vi "Save Layout.vi"(5 "MultiPlotPanel in":refnum<class "MultiPlotPanel.lvclass">, 8 "error in (no error)":errorcluster, 10 "file extension":string, 11 "Loop data in":T1 {"PanelMap"."Data"."Plot Bounds (%)"."Bottom (%)" format="%.2f"; "PanelMap"."Data"."Plot Bounds (%)"."Top (%)" format="%.2f"; "PanelMap"."Data"."Plot Bounds (%)"."Right (%)" format="%.2f"; "PanelMap"."Data"."Plot Bounds (%)"."Left (%)" format="%.2f"}) -> (0 "error out":errorcluster, 1 "Valid save?":bool, 2 "Filename":string, 3 "Loop data out":T1 {"PanelMap"."Data"."Plot Bounds (%)"."Bottom (%)" format="%.2f"; "PanelMap"."Data"."Plot Bounds (%)"."Top (%)" format="%.2f"; "PanelMap"."Data"."Plot Bounds (%)"."Right (%)" format="%.2f"; "PanelMap"."Data"."Plot Bounds (%)"."Left (%)" format="%.2f"})   [LabVIEW 2021, in "MultiStokePlot.lvlib" / "MultiPlotPanel.lvclass"]
uses:
  Classes/MultiPlotPanel/MultiPlotPanel.lvclass
  Loop Data.ctl
  <vilib>/IlluminatedG/IG OOPanel/OOPanel/Manager/Manager.lvclass
  Panel Map.ctl
  Panel Map Data.ctl
  <userlib>/bjustice/RocketPlot/Classes/RocketPlotPanel/RocketPlotPanel.lvclass
  Window Position.ctl
  <vilib>/IlluminatedG/IG OOPanel/OOPanel/Panel/Panel Events.ctl
  <vilib>/IlluminatedG/IG OOPanel/OOPanel/Panel/Visbility Event Data.ctl
  <vilib>/IlluminatedG/IG OOPanel/OOPanel/Visibility State.ctl
  <vilib>/IlluminatedG/IG OOPanel/OOPanel/Close Reason.ctl
  Classes/MultiPlotPanel/MultiPlotPanel.lvclass/MultiPlotPanel.ctl
  Classes/BlueMultiPlotConfig/SinglePlotConfig.ctl
  <userlib>/bjustice/RocketPlot/TypeDefs/plot load data V2.ctl
  <userlib>/bjustice/RocketPlot/TypeDefs/plot properties V2.ctl
  <userlib>/bjustice/RocketPlot/TypeDefs/plot attributes V2.ctl
  <userlib>/bjustice/RocketPlot/TypeDefs/Plot scale axis properties.ctl
  <userlib>/bjustice/RocketPlot/TypeDefs/Plot general properties.ctl
  <userlib>/bjustice/RocketPlot/Classes/RocketPlotPanel/RocketPlotPanel.lvclass/RocketPlotPanel.ctl
  <userlib>/bjustice/RocketPlot/Classes/RocketPlotPanel/Read RocketPlotHandle.vi
  <userlib>/bjustice/RocketPlot/Classes/RocketPlotHandle/RocketPlotHandle.lvclass
  <userlib>/bjustice/RocketPlot/RocketPlot.lvlib
  <vilib>/IlluminatedG/IG OOPanel/OOPanel/OOPanel.lvlib
  <vilib>/IlluminatedG/IG OOPanel/OOPanel/Panel/Panel.lvclass
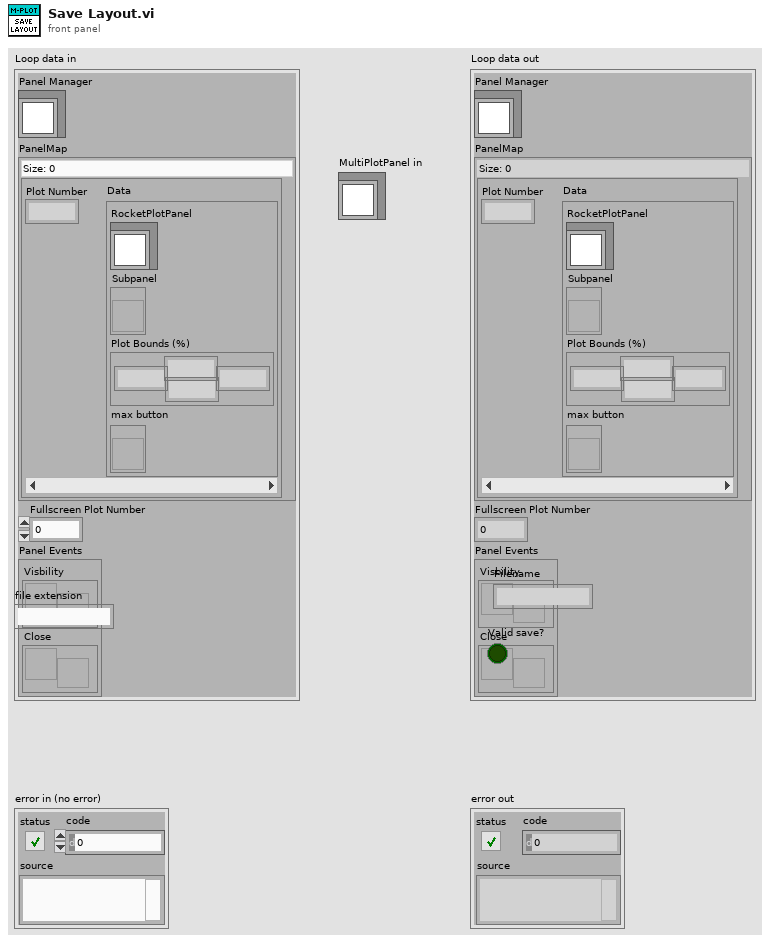
[diagram p1: front panel]
types:
  T1 = typedef "MultiStokePlot.lvlib/MultiPlotPanel.lvclass/Loop Data.ctl" = cluster{"Panel Manager":refnum<class "Manager.lvclass">, "PanelMap":T2, "Fullscreen Plot Number":i32, "Panel Events":T5}
  T2 = typedef "MultiStokePlot.lvlib/MultiPlotPanel.lvclass/Panel Map.ctl" = map{i32, T3}
  T3 = typedef "MultiStokePlot.lvlib/MultiPlotPanel.lvclass/Panel Map Data.ctl" = cluster{"RocketPlotPanel":refnum<class "RocketPlotPanel.lvclass">, "Subpanel":refnum<vi>, "Plot Bounds (%)":T4, "max button":refnum<vi>}
  T4 = typedef "MultiStokePlot.lvlib/MultiPlotPanel.lvclass/Window Position.ctl" = cluster{"Left (%)":dbl, "Top (%)":dbl, "Right (%)":dbl, "Bottom (%)":dbl}
  T5 = typedef "OOPanel.lvlib/Panel.lvclass/Panel Events.ctl" = cluster{"Visbility":refnum<user-event>, "Close":refnum<user-event>}
  T6 = typedef "MultiStokePlot.lvlib/MultiPlotPanel.lvclass/SinglePlotConfig.ctl" = cluster{"Plot Number":i32, "Plot Bounds (%)":T4, "RocketPlotConfig":T7}
  T7 = typedef "RocketPlot.lvlib/plot load data V2.ctl" = cluster{"plots":T8[], "X-axis":T10, "Y-axes":T10[], "General":T11}
  T8 = typedef "RocketPlot.lvlib/plot properties V2.ctl" = cluster{"attributes":T9, "Numeric":dbl, "Flatline?":bool}
  T9 = typedef "RocketPlot.lvlib/plot attributes V2.ctl" = cluster{"Plot Color":u32, "Point Style":u8, "Line Style":u8, "Plot Interpolation":u8, "Line Width":u8, "Bar Plot Style":u8, "Fill To":i16, "X Scale Index":u32, "Y Scale Index":u32, "Anti-aliased":bool, "Label Format":u8, "Digital Transition Type":u8, "Digital Transition Location":u8, "Digital Line Style":u8, "Fill/Point Color":u32, "Plot Name":string, "Visible":bool}
  T10 = typedef "RocketPlot.lvlib/Plot scale axis properties.ctl" = cluster{"Name Label.Text":string, "Style":u8, "Tick Colors:Minor Tick Color":u32, "Tick Colors:Tick Color":u32, "Marker Colors:Text Color":u32, "Grid Colors:Major Color":u32, "Grid Colors:Minor Color":u32, "Mapping Mode":u8, "Flipped":bool, "Name Label.Visible":bool, "Name Label.Text Colors:Text Color":u32, "Scale Fit":u8, "Range:Maximum":dbl, "Range:Minimum":dbl, "Offset and Multiplier:Multiplier":dbl, "Offset and Multiplier:Offset":dbl, "Name Label.Font:Size":u32, "Marker.Font:Size":u32, "Uniform Marker Spacing?":bool, "Format String":string}
  T11 = typedef "RocketPlot.lvlib/Plot general properties.ctl" = cluster{"Title":string, "Time to Plot":dbl, "Title.Visible":bool, "Sidebar.Visible":bool, "Plot Area:Colors:BG Color":u32, "X Scale.Plot Name":string, "X Scale.Use Plot Name":bool}
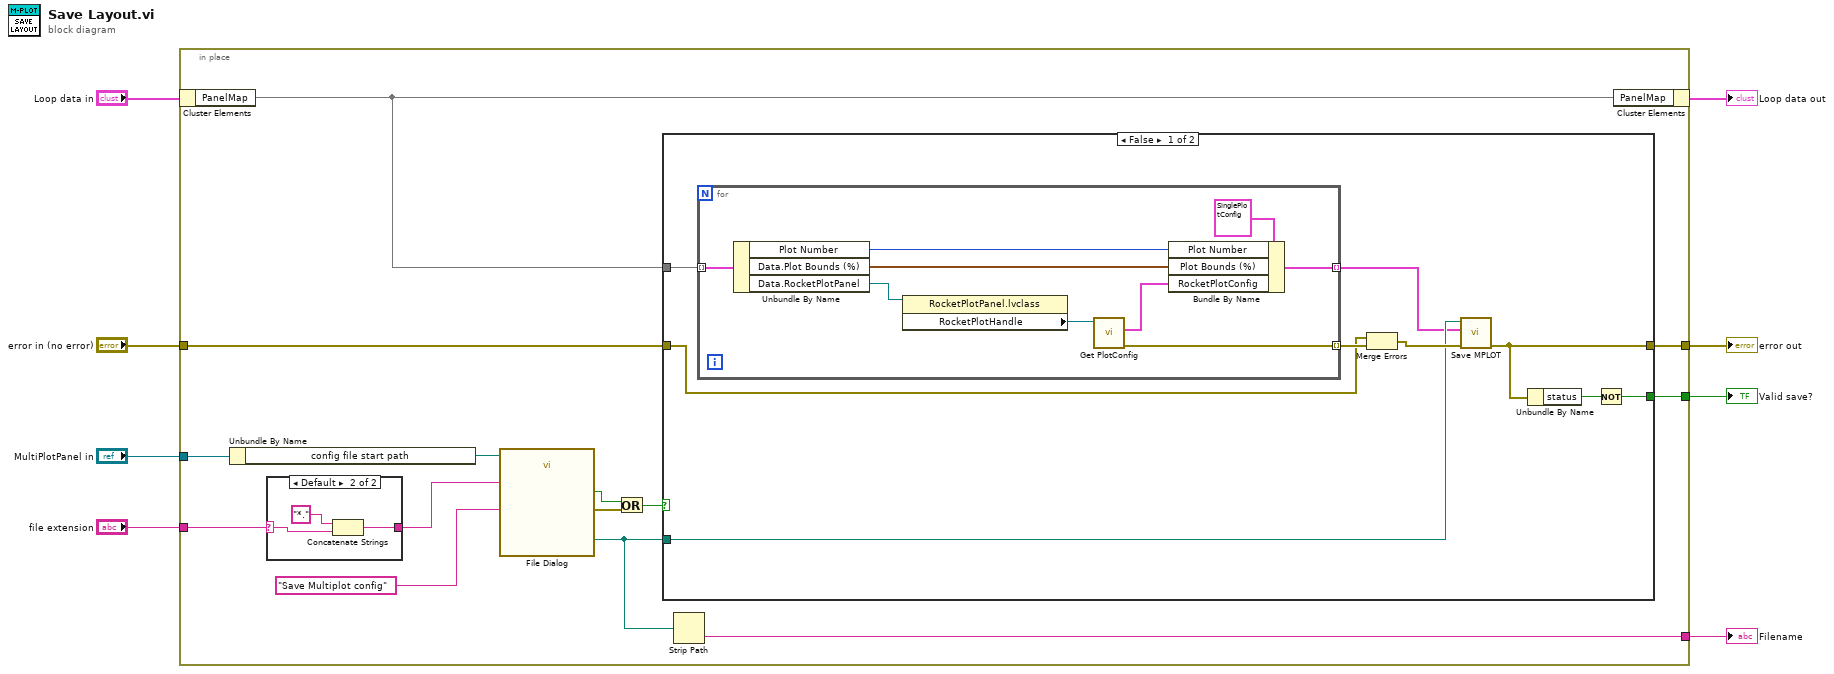
[diagram p0: block diagram]
diagram:
  n1 = in-place {
    in-place-border: "error in (no error)" -> [w14]
    in-place-border: "file extension" -> [w18]
    in-place-border: [w15] -> w4
    in-place-border: "MultiPlotPanel in" -> [w13]
    in-place-border: [w10] -> w2
    in-place-border: [w9] -> w1
    n2 = in-place-cluster #1("Loop data in") -> ("PanelMap"=w16:T2)
    n3 = Unbundle By Name(w13) -> ("config file start path"=w12:path)
    n4 = case shown="Default" w18 {
      selector: w18 -> [w42 w44]
      tunnel: [w42 w43] -> w22
      frame "" {
      }
      frame Default {
        n5 = Concatenate Strings("*." ("string"), w44) -> (w43:string)
      }
    }
    n6 = call "File Dialog"("start path"=w12, "prompt"="Save Multiplot config", "pattern (all files)"=w22) -> ("selected path"=w11:path, "cancelled"=w20:bool, "error out"=w19:errorcluster)  [unwired: 9 in, 1 out]
    n7 = Or(x=w20, y=w19) -> (x .or. y?=w17:bool)
    n8 = case shown="False" w17 {
      tunnel: w16 -> [w31 _]
      tunnel: w11 -> [w24 _]
      tunnel: [w27 w41] -> w15
      tunnel: w14 -> [w28 w41]
      tunnel: [w25 _] -> w9
      frame False {
        n9 = for {
          tunnel: w31 -> [w39] mode=indexing
          tunnel: [w34] -> w23 mode=indexing
          tunnel: [w32] -> w30 mode=indexing
          n10 = Unbundle By Name(w39) -> ("Plot Number"=w38:i32, "Data.Plot Bounds (%)"=w35:T4, "Data.RocketPlotPanel"=w37:refnum<class "RocketPlotPanel.lvclass">)
          n11 = property class="RocketPlotPanel.lvclass"(reference=w37) -> ("RocketPlotHandle"=w36:refnum<class "RocketPlotHandle.lvclass">)  [unwired: 1 in, 2 out]
          n12 = call <userlib>:"Get PlotConfig.vi"("BluePlotHandle in"=w36) -> ("error out"=w32:errorcluster, "Plot config"=w33:T7)  [unwired: 8 in, 1 out]
          n13 = Bundle By Name(cluster=T6 {"Plot Number"=0, "Plot Bounds (%)"={"Left (%)"=0.0, "Top (%)"=0.0, "Right (%)"=0.0, "Bottom (%)"=0.0}, "RocketPlotConfig"={"plots"=[], "X-axis"={"Name Label.Text"="", "Style"=0, "Tick Colors:Minor Tick Color"=0, "Tick Colors:Tick Color"=0, "Marker Colors:Text Color"=0, "Grid Colors:Major Color"=0, "Grid Colors:Minor Color"=0, "Mapping Mode"=0, "Flipped"=FALSE, "Name Label.Visible"=FALSE, "Name Label.Text Colors:Text Color"=0, "Scale Fit"=0, "Range:Maximum"=0.0, "Range:Minimum"=0.0, "Offset and Multiplier:Multiplier"=0.0, "Offset and Multiplier:Offset"=0.0, "Name Label.Font:Size"=0, "Marker.Font:Size"=0, "Uniform Marker Spacing?"=TRUE, "Format String"=""}, "Y-axes"=[], "General"={"Title"="", "Time to Plot"=1800.0, "Title.Visible"=FALSE, "Sidebar.Visible"=FALSE, "Plot Area:Colors:BG Color"=0, "X Scale.Plot Name"="", "X Scale.Use Plot Name"=FALSE}}} ("Cluster"), "Plot Number"=w38, "Plot Bounds (%)"=w35, "RocketPlotConfig"=w33) -> (w34:T6)
        }
        n14 = Merge Errors(w28, w30) -> (w29:errorcluster)
        n15 = call "Save MPLOT.vi"("error in (no error)"=w29, "RocketPlots"=w23, "Filepath"=w24) -> ("error out"=w27:errorcluster)  [unwired: 8 in]
        n16 = Unbundle By Name(w27) -> ("status"=w26:bool)
        n17 = Not(x=w26) -> (.not. x?=w25:bool)
      }
      frame True {
      }
    }
    n18 = Strip Path(path=w11) -> (name=w10:string)  [unwired: 1 out]
    n19 = in-place-cluster #1("PanelMap"=w16) -> (→"Loop data out":T1)
  }
  "error out" <- w4
  "Filename" <- w2
  "Valid save?" <- w1
